vi "InputPadRef.vi"() -> ()   [LabVIEW 2012, in "StimulCtrls.lvlib"]
uses:
  StimulCtrls.lvlib
panel:
  in  "NumControl":refnum<vi>
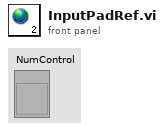
[diagram p1: front panel]
diagram:
